vi "WD Polling.vi"() -> ()   [LabVIEW 2015]
doc: "This VI creates an FPGA personality to emulate a hardware watchdog. If the whack control is not asserted prior to a software-defined expiration (in milliseconds), an indicator will show that the watchdog has timed out. For the sbRIO evaluation board, the Armed control is set to SWITCH1 and the Whack control is set to PB1."
uses:
  <vilib>/Platform/TimedLoop/XDataNode/timing_clust.ctl
  <vilib>/Platform/TimedLoop/XDataNode/nitl_modes.ctl
  <vilib>/Platform/TimedLoop/XDataNode/wakeup.ctl
  Instance           1 20Saved   WD - Polling .vi
  <vilib>/rvi/Emulation/niFpgaSctlEmulationGetInTimedLoop.vi
  <vilib>/rvi/Emulation/niFpgaEmulationReportErrorSimple.vi
  <vilib>/rvi/Emulation/niFpgaGetClockAttributes.vi
  <vilib>/rvi/Emulation/niFpgaCriticalErrorInLSC.vi
  <vilib>/rvi/eio/common/nirviEmuTemplateMethod_errors.vi
  <vilib>/Platform/TimedLoop/XDataNode/XDataNode.xnode
  <vilib>/eio/EIONode/EIONode.xnode
  <vilib>/Platform/TimedLoop/XDataNode/XDNodeRunTimeDep.lvlib
panel:
  out "Whack":bool
  out "Armed":bool
  in  "Timeout (ms)":u32=1000
  in  "stop":bool
  out "Expired":bool
  # "This FPGA VI emulates a hardware watchdog. If the whack control is not \nasserted prior to a software-defined expiration (in milliseconds), an \nindicator will show that the watchdog has expired. For the evaluation board,\nthe physical Armed control is PB1 and the Whack control is PB2. Press PB1 then PB2 to Whack the watchdog before the Timeout period, else the timer expires. If you change the timeout period, rearm the watchdog. In an actual application, the Whack functionality would be in a processor loop."
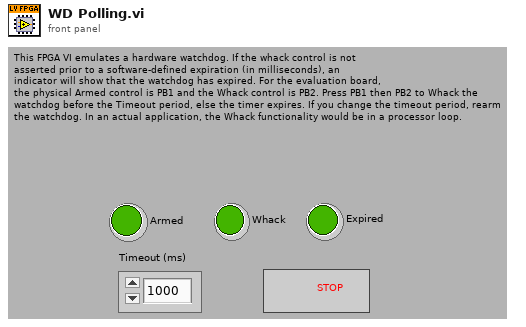
[diagram p1: front panel]
types:
  T1 = typedef "XDNodeRunTimeDep.lvlib/timing_clust.ctl" = cluster{"Expected End [f-1]":u64, "Actual End [f-1]":u64, "Finished Late? [f-1]":bool, "Expected End [i-1]":u64, "Actual End [i-1]":u64, "Finished Late? [i-1]":bool, "Expected Start [i]":u64, "Actual Start [i]":u64, "Expected Start [f]":u64, "Actual Start [f]":u64, "Source Name":string, "Structure Name":string, "Period":i64, "Deadline":i64, "Offset":i64, "Start":i64, "Priority":i32, "Timeout":i32, "Mode":T2, "Wakeup Reason":T3, "Error":errorcluster, "Source Type":string, "Secondary Source Type":string, "Global End Time":u64, "Global Start Time":u64, "Frame Duration":u64, "Iteration Duration":u64, "Assigned CPU":i32, "I/O Scan Engine Mode":u32}
  T2 = typedef "XDNodeRunTimeDep.lvlib/nitl_modes.ctl" = enum32{"No Change", "Process missed periods, maintain original phase", "Discard missed periods, maintain original phase", "Process missed periods, ignore original phase", "Discard missed periods, ignore original phase"}
  T3 = typedef "XDNodeRunTimeDep.lvlib/wakeup.ctl" = enum32{"Normal", "Aborted", "Asynchronous wakeup", "Timing source error", "Timed loop error", "Timeout"}
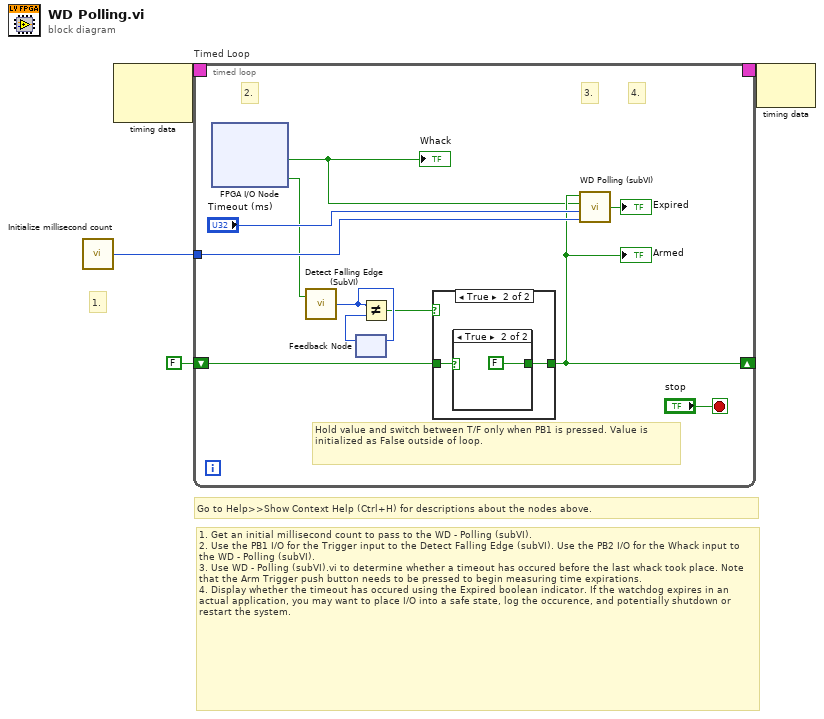
[diagram p0: block diagram]
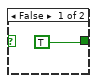
[diagram p3: hidden frame]
diagram:
  # "Go to Help>>Show Context Help (Ctrl+H) for descriptions about the nodes above."
  # "1."
  # "1. Get an initial millisecond count to pass to the WD - Polling (subVI).\n2. Use the PB1 I/O for the Trigger input to the Detect Falling Edge (subVI). Use the PB2 I/O for the Whack input to the WD - Polling (subVI).\n3. Use WD - Polling (subVI).vi to determine whether a timeout has occured before the last whack took place. Note that the Arm Trigger push button needs to be pressed to begin measuring time expirations.\n4. Display whether the timeout has occured using the Expired boolean indicator. If the watchdog expires in an actual application, you may want to place I/O into a safe state, log the occurence, and potentially shutdown or restart the system."
  n1 = call "Initialize millisecond count"() -> ("Tick Count(mSec)"=w2:u32)
  n2 = node-c288() -> (w3:T1)  [unwired: 2 out]
  n3 = timed-loop "Timed Loop" {
    timing-out: [_] -> w4
    timing: w3 -> [_]
    tunnel: w2 -> [w14]
    shift-right: [w7] -> _
    shift-left: FALSE -> [w8]
    stop <- "stop" stop-if-true
    # "Hold value and switch between T/F only when PB1 is pressed. Value is initialized as False outside of loop."
    # "4."
    # "3."
    # "2."
    n4 = xnode "FPGA I/O Node"() -> ("PB2"=w5:bool, "PB1"=w6:bool)  [unwired: 2 in, 2 out]
    "Whack" <- w5
    n5 = call "Detect Falling Edge (SubVI).vi"("Trigger"=w6) -> ("8-bit Count (0-63)"=w10:u8)  [unwired: 1 in]
    n6 = feedback-in #1(w10) -> ()
    n7 = feedback #1() -> (w11:u8)  [unwired: 1 in]
    n8 = Not Equal?(x=w10, y=w11) -> (x != y?=w9:bool)
    n9 = case shown="True" w9 {
      tunnel: w8 -> [w16 w18]
      tunnel: [w16 w17] -> w7
      frame False {
      }
      frame True {
        n10 = case shown="True" w18 {
          tunnel: [TRUE FALSE] -> w17
          frame False {
          }
          frame True {
          }
        }
      }
    }
    "Armed" <- w7
    n11 = call "WD Polling (subVI).vi"("Timer Initialize (ms)"=w14, "Timeout (ms)"="Timeout (ms)", "Whack"=w5, "Arm"=w7) -> ("Expired"=→"Expired":bool)  [unwired: 2 out]
  }
  n12 = node-c288(w4) -> ()  [unwired: 1 out]
